vi "Get Max add 1 from num string.vi"(11 "Input Array":string[](array[string])) -> (2 "Max":string, 3 "Max Num +1":string)   [LabVIEW 2021]
doc: "when select from DB, delete duplite elements, and get max ,+1.\n2016-09-06 15:30:51\n蒋松\nsina：@sushu1051"
panel:
  out "indices of removed elements":i32[](array[numeric])
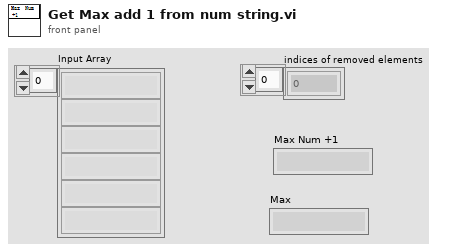
[diagram p1: front panel]
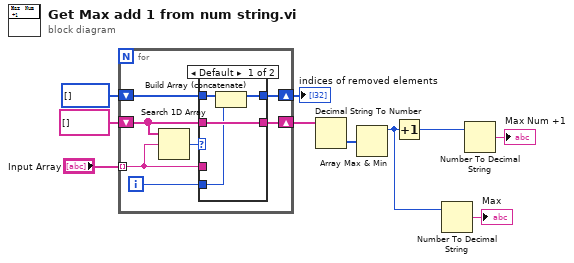
[diagram p0: block diagram]
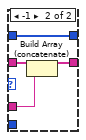
[diagram p2: hidden frame]
diagram:
  n1 = for {
    tunnel: "Input Array" -> [w16] mode=indexing
    shift-right: [w15] -> w4
    shift-left: string[] [] -> [w14]
    shift-right: [w12] -> w8
    shift-left: i32[] [] -> [w11]
    i -> [w13]
    n2 = Search 1D Array(1D array=w14, element=w16) -> (index of element=w17:i32)  [unwired: 1 in]
    n3 = case shown="Default" w17 {
      tunnel: w16 -> [_ w25]
      tunnel: [w21 w23] -> w15
      tunnel: w14 -> [w21 w24]
      tunnel: w13 -> [w18 _]
      tunnel: [w19 w22] -> w12
      tunnel: w11 -> [w20 w22]
      frame Default {
        n4 = Build Array (concatenate)(w20, w18) -> (w19:i32[])
      }
      frame -1 {
        n5 = Build Array (concatenate)(w24, w25) -> (w23:string[])
      }
    }
  }
  "indices of removed elements" <- w8
  n6 = Decimal String To Number(string=w4) -> (number=w9:i32[])  [unwired: 2 in, 1 out]
  n7 = Array Max & Min(array=w9) -> (max value=w2:i32)  [unwired: 3 out]
  n8 = Increment(x=w2) -> (x+1=w10:i32)
  n9 = Number To Decimal String(number=w2) -> (decimal integer string=→"Max":string)  [unwired: 1 in]
  n10 = Number To Decimal String(number=w10) -> (decimal integer string=→"Max Num +1":string)  [unwired: 1 in]
